vi "Logarithm Fit.vi"(0 "Y":dbl[](array[numeric]), 1 "base":dbl(ring)=2.71828 items=["e"=2.71828, "2"=2.0, "10"=10.0], 5 "X":dbl[](array[numeric]), 7 "Weight":dbl[](array[numeric]), 9 "tolerance":dbl=0.0001 format="%#_3g", 11 "method":T2 items=["Least Square", "Least Absolute Residual", "Bisquare"], 12 "parameter bounds":T1={"amp min"=-inf, "amp max"=inf, "scale min"=-inf, "scale max"=inf}) -> (4 "Best Logarithm Fit":dbl[](array[numeric]), 6 "amplitude":dbl, 8 "scale":dbl, 14 "residue":dbl, 15 "error":i32)   [LabVIEW 2017, in "NI_AALPro.lvlib"]
doc: "Returns the logarithmic fit of a data set (<B>X</B>, <B>Y</B>) using the Least Square, Least Absolute Residual, or Bisquare method."
uses:
  <vilib>/Analysis/NI_AALPro.lvlib
  <vilib>/Analysis/6fits.llb/Curve Fitting Criteria.ctl
  <resource>/lvanlys.dll
panel:
  # "Constrained Logarithm Fit"
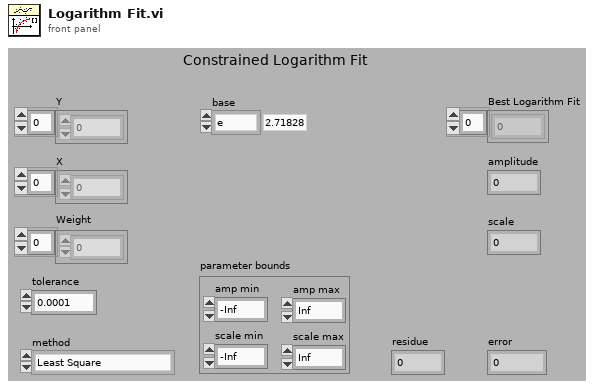
[diagram p1: front panel]
types:
  T1 = cluster{"amp min":dbl, "amp max":dbl, "scale min":dbl, "scale max":dbl}
  T2 = typedef "NI_AALPro.lvlib/Curve Fitting Criteria.ctl" = u16
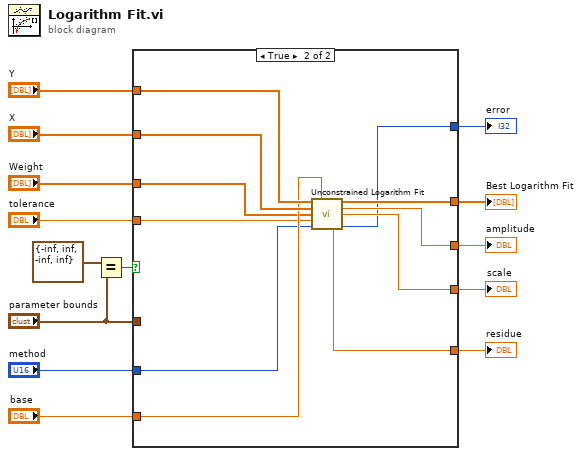
[diagram p0: block diagram]
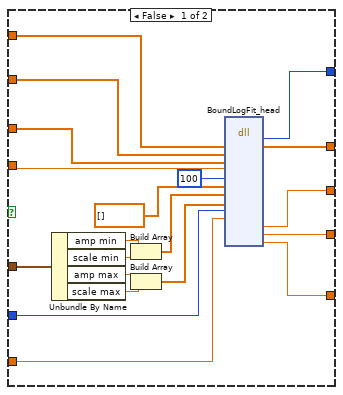
[diagram p2: hidden frame]
diagram:
  n1 = Equal?(x=T1 {"amp min"=-inf, "amp max"=inf, "scale min"=-inf, "scale max"=inf} ("parameter bounds 2"), y="parameter bounds") -> (x = y?=w3:bool)
  n2 = case shown="True" w3 {
    tunnel: "Y" -> [w34 w45]
    tunnel: "X" -> [w33 w44]
    tunnel: "Weight" -> [w32 w37]
    tunnel: "tolerance" -> [w31 w36]
    tunnel: "method" -> [w28 w35]
    tunnel: [w27 w43] -> w9
    tunnel: [w26 w42] -> w8
    tunnel: [w25 w41] -> w7
    tunnel: [w24 w40] -> w6
    tunnel: "base" -> [w23 w38]
    tunnel: "parameter bounds" -> [w22 _]
    tunnel: [w15 w39] -> w4
    frame False {
      n3 = Unbundle By Name(w22) -> ("amp min"=w21:dbl, "scale min"=w20:dbl, "amp max"=w19:dbl, "scale max"=w18:dbl)
      n4 = Build Array(w21, w20) -> (w17:dbl[])
      n5 = Build Array(w19, w18) -> (w16:dbl[])
      n6 = dll-call lib="e:/builds/penguin/labview/branches/2017/dev/dist/resource/lvanlys.*" fn="BoundLogFit_head"("y"=w34, "x"=w33, "weight"=w32, "tolerance"=w31, "maxIter"=100, "intial coef"=dbl[] [] ("initial coefficients"), "minBound"=w17, "maxBound"=w16, "algorithm"=w28, "base"=w23) -> ("return type"=w24:i32, "y"=w27:dbl[], "amp"=w26:dbl, "power"=w25:dbl, "residue"=w15:dbl)  [unwired: 10 in, 7 out]
    }
    frame True {
      n7 = call <vilib>:"Unconstrained Logarithm Fit.vi"("Y"=w45, "base"=w38, "X"=w44, "Weight"=w37, "tolerance"=w36, "method"=w35) -> ("Best Logarithm Fit"=w43:dbl[], "amplitude"=w42:dbl, "scale"=w41:dbl, "residue"=w39:dbl, "error"=w40:i32)  [unwired: 5 out]
    }
  }
  "scale" <- w7
  "amplitude" <- w8
  "Best Logarithm Fit" <- w9
  "error" <- w6
  "residue" <- w4
